vi "getType.vi"(8 "error in (no error)":errorcluster, 11 "Loop in":refnum<class "Loop.lvclass">) -> (0 "error out":errorcluster, 2 "type":enum16{"Point", "Loop", "Scan"}(ring), 3 "Loop out":refnum<class "Loop.lvclass">)   [LabVIEW 2011, in "Tools.lvlib" / "Sequencing.lvlib" / "Loop.lvclass"]
uses:
  Loop.lvclass
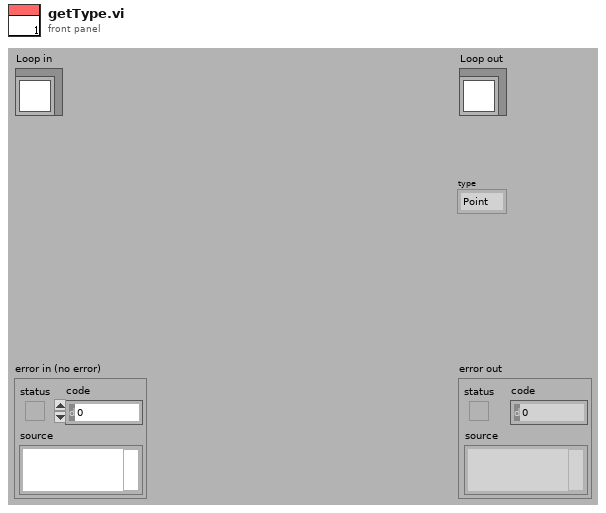
[diagram p1: front panel]
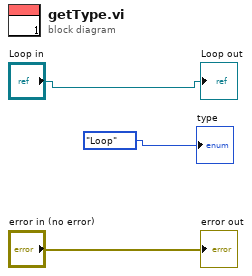
[diagram p0: block diagram]
diagram:
  "error out" <- "error in (no error)"
  "Loop out" <- "Loop in"
  "type" <- enum16{"Point", "Loop", "Scan"}."Loop" ("type")
